vi "data_calibrate_and_grid.vi"(6 "Reset":bool=TRUE, 8 "Tare":bool=TRUE, 9 "Row Length":i32=64, 10 "No. Nodes":i32=64, 11 "Sensor Readings (PACKET)":i16[](array[numeric])) -> (0 "Node XYZ List":dbl[][](array[numeric]), 1 "Y (GRID)":dbl[][](array[numeric]), 2 "X (GRID)":dbl[][](array[numeric]), 3 "Z (GRID)":dbl[][](array[numeric]), 4 "Mag_GRID":dbl[][](array[numeric]))   [LabVIEW 2018]
panel:
  in  "Position Gain":dbl[](array[numeric])=[0.005, 0.005, 0.001]
  in  "Y Coords":dbl[](array[numeric])=[0.0, 15.0, 30.0, 45.0, 60.0, 75.0, 90.0, 105.0]
  in  "X Coords":dbl[](array[numeric])=[0.0, 15.0, 30.0, 45.0, 60.0, 75.0, 90.0, 105.0]
  in  "Tab Control":enum32{"16 Node", "64 Node"}(tab)=enum."64 Node"
  in  "Lookup Index n16":i32[](array[numeric])=[0, 2, 1, 3, 4, 6, 5, 7, 8, 10, 9, 11, 12, 14, 13, 15]
  in  "Inv Gain n16":i32[][](array[numeric])=[[1, 1, 1], [1, 1, -1], [1, 1, 1], [1, 1, 1], [1, 1, 1], [1, 1, -1], [1, 1, -1], [1, 1, -1], [1, 1, -1], [1, 1, -1], [1, 1, -1], [1, 1, 1], [1, 1, -1], [1, 1, 1], [1, 1, 1], [1, 1, -1]]
  in  "Lookup Index n64":i32[](array[numeric])=[0, 1, 2, 3, 4, 5, 6, 7, 15, 14, 13, 12, 11, 10, 9, 8, 16, 17, 18, 19, 20, 21, 22, 23, 31, 29, 30, 28, 27, 26, 25, 24, 32, 33, 34, 35, 36, 37, 38, 39, 47, 46, 45, 44, 43, 42, 41, 40, 55, 54, 53, 52, 51, 50, 49, 48, 63, 62, 61, 60, 59, 58, 57, 56]
  in  "Inv Gain n64":i32[][](array[numeric])=[[1, 1, 1], [1, 1, 1], [1, 1, 1], [1, 1, 1], [1, 1, 1], [1, 1, 1], [1, 1, 1], [1, 1, 1], [1, 1, 1], [1, 1, 1], [1, 1, 1], [1, 1, 1], [1, 1, 1], [1, 1, 1], [1, 1, 1], [1, 1, 1], [1, 1, 1], [1, 1, 1], [1, 1, 1], [1, 1, 1], [1, 1, 1], [1, 1, 1], [1, 1, 1], [1, 1, 1], [1, 1, 1], [1, 1, 1], [1, 1, -1], [1, 1, 1], [1, 1, 1], [1, 1, 1], [1, 1, 1], [1, 1, 1], [1, 1, 1], [1, 1, 1], [1, 1, 1], [1, 1, 1], [1, 1, 1], [1, 1, 1], [1, 1, 1], [1, 1, 1], [1, 1, 1], [1, 1, 1], [1, 1, 1], [1, 1, 1], [1, 1, 1], [1, 1, 1], [1, 1, 1], [1, 1, 1], [1, 1, 1], [1, 1, 1], [1, 1, 1], [1, 1, 1], [1, 1, 1], [1, 1, 1], [1, 1, 1], [1, 1, 1], [1, 1, 1], [1, 1, 1], [1, 1, 1], [1, 1, -1], [1, 1, -1], [1, 1, 1], [1, 1, 1], [1, 1, 1]]
  in  "Tare":dbl[][](array[numeric])=[[0.00018775, -0.000174232, 3312.98], [0.000139686, -0.00039953199999999997, 2906.42], [-0.000288384, -0.001229387, 2606.34], [-3.6799e-05, -0.0012016, 3702.6], [0.000266605, -0.001108476, 3847.7999999999997], [0.00038301, -0.000208027, 3472.7], [-0.000177236, -0.000316171, 3651.7799999999997], [-0.00024557699999999997, 0.000544475, 4767.4], [-5.6325e-05, -0.00041305, 4172.08], [8.4112e-05, 0.000956774, 2562.7799999999997], [-0.000261348, 0.001097962, 3675.98], [-0.00014944899999999998, -0.00066839, 4856.94], [-0.000204272, 0.000920726, 4740.78], [-0.000242573, -7.7353e-05, 4009.94], [0.000246328, -0.000138184, 4358.42], [7.51e-06, 0.000451351, 5829.78]]
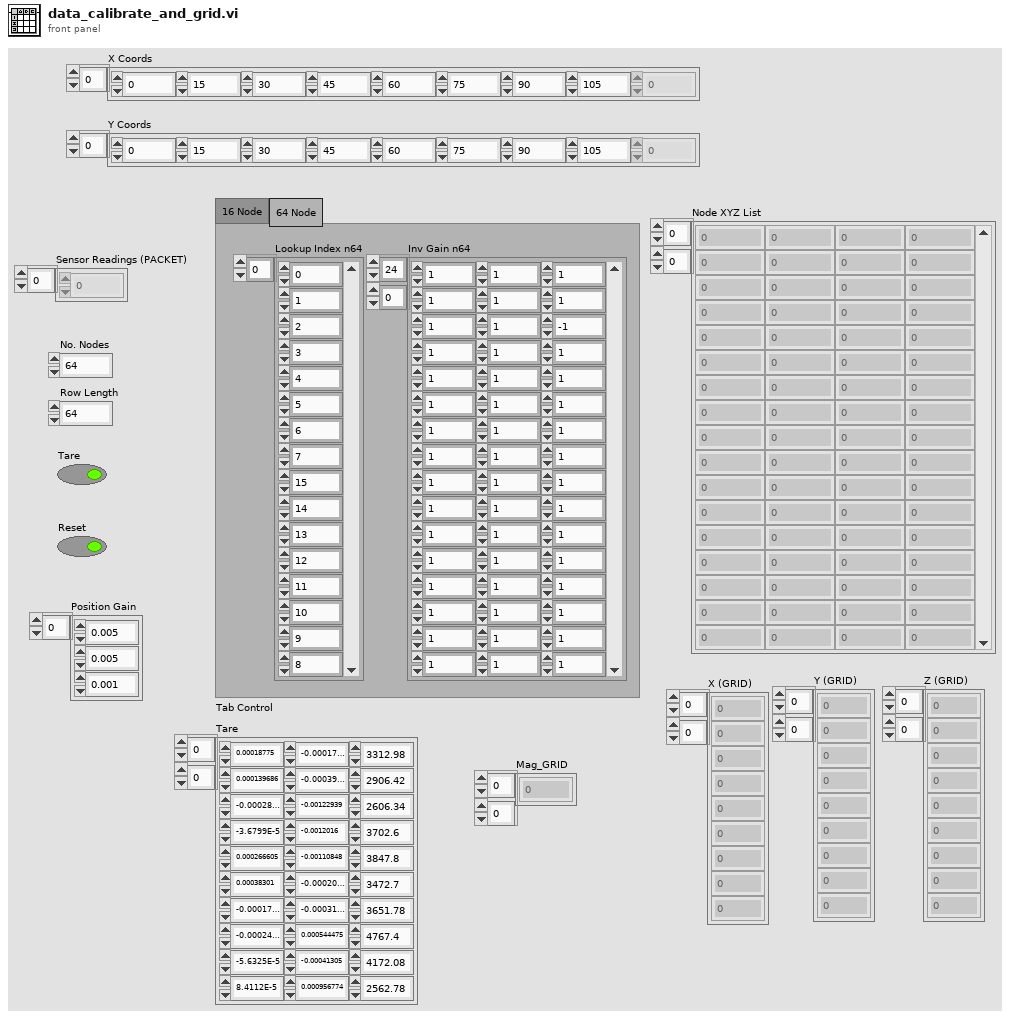
[diagram p1: front panel]
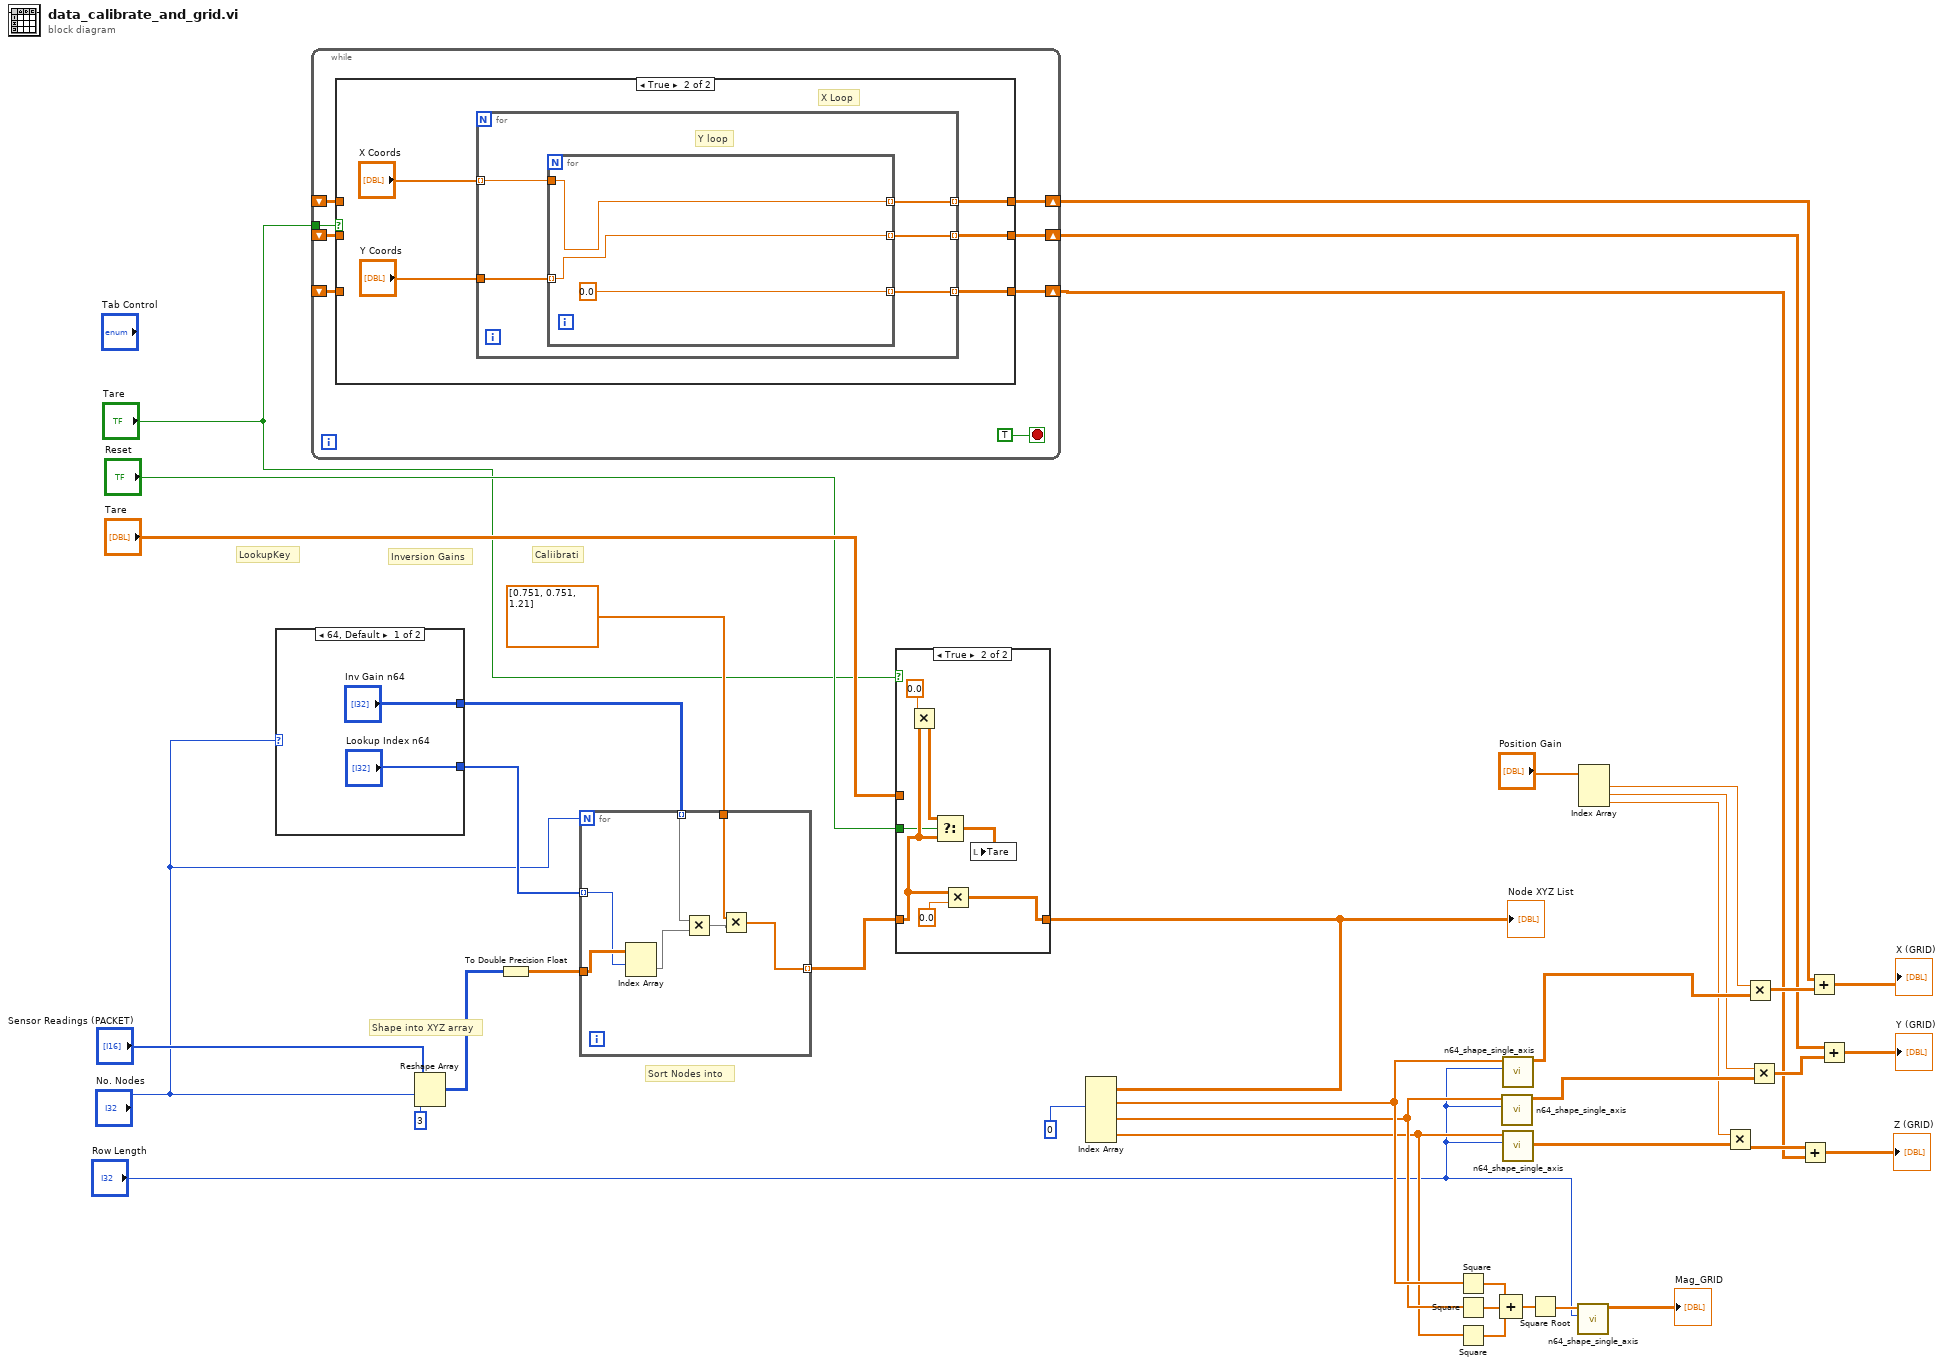
[diagram p0: block diagram]
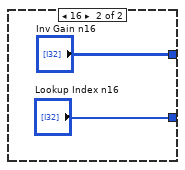
[diagram p3: hidden frame]
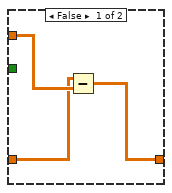
[diagram p4: hidden frame]
diagram:
  # "Caliibrati"
  # "Inversion Gains"
  # "LookupKey"
  # "Sort Nodes into"
  # "Shape into XYZ array"
  n1 = case shown="64, Default" "No. Nodes" {
    tunnel: ["Lookup Index n64" "Lookup Index n16"] -> w37
    tunnel: ["Inv Gain n64" "Inv Gain n16"] -> w35
    frame 64, Default {
    }
    frame 16 {
    }
  }
  n2 = while {
    tunnel: "Tare" -> [w52]
    shift-right: [w50] -> w12
    shift-left: _ -> [w47]
    shift-right: [w49] -> w9
    shift-left: _ -> [w46]
    shift-right: [w48] -> w2
    shift-left: _ -> [w45]
    stop <- TRUE stop-if-true
    n3 = case shown="True" w52 {
      tunnel: [w55 w58] -> w50
      tunnel: [w54 w57] -> w49
      tunnel: [w53 w56] -> w48
      tunnel: w47 -> [w55 _]
      tunnel: w46 -> [w54 _]
      tunnel: w45 -> [w53 _]
      frame False {
      }
      frame True {
        # "X Loop"
        n4 = for {
          tunnel: "X Coords" -> [w65] mode=indexing
          tunnel: "Y Coords" -> [w64]
          tunnel: [w63] -> w58 mode=indexing
          tunnel: [w62] -> w56 mode=indexing
          tunnel: [w61] -> w57 mode=indexing
          # "Y loop"
          n5 = for {
            tunnel: w65 -> [w68]
            tunnel: w64 -> [w66] mode=indexing
            tunnel: [w68] -> w63 mode=indexing
            tunnel: [0.0 ("element")] -> w62 mode=indexing
            tunnel: [w66] -> w61 mode=indexing
          }
        }
      }
    }
  }
  n6 = Reshape Array("Sensor Readings (PACKET)", "No. Nodes", 3 ("milliseconds to wait")) -> (w34:i16[][])
  n7 = To Double Precision Float(number=w34) -> (double precision float=w33:dbl[][])
  n8 = for {
    N: "No. Nodes" -> [_]
    tunnel: w33 -> [w75]
    tunnel: w37 -> [w69] mode=indexing
    tunnel: [w70] -> w32 mode=indexing
    tunnel: dbl[] [0.751, 0.751, 1.21] -> [w72]
    tunnel: w35 -> [w74] mode=indexing
    n9 = Index Array(array=w75, index (row)=w69) -> (element=w71:dbl[])  [unwired: 1 in]
    n10 = Multiply(x=w74, y=w71) -> (x*y=w73:dbl[])
    n11 = Multiply(x=w72, y=w73) -> (x*y=w70:dbl[])
  }
  n12 = case shown="True" "Tare" {
    tunnel: w32 -> [w76 w82]
    tunnel: [w78 w84] -> w31
    tunnel: "Tare" -> [w77 _]
    tunnel: "Reset" -> [_ w79]
    frame False {
      n13 = Subtract(x=w76, y=w77) -> (x-y=w78:dbl[][])
    }
    frame True {
      n14 = Multiply(x=0.0 ("milliseconds to wait"), y=w82) -> (x*y=w81:dbl[][])
      n15 = Select(t=w81, s=w79, f=w82) -> (s? t:f=w83:dbl[][])
      n16 = Multiply(x=w82, y=0.0 ("milliseconds to wait")) -> (x*y=w84:dbl[][])
      n17 = local write "Tare"(w83) -> ()
    }
  }
  "Node XYZ List" <- w31
  n18 = Index Array(array=w31, index (col) #1=0 ("disabled index (col)")) -> (element #1=w28:dbl[], element #2=w27:dbl[], element #3=w26:dbl[])  [unwired: 5 in]
  n19 = Square(x=w28) -> (x^2=w25:dbl[])
  n20 = Square(x=w27) -> (x^2=w23:dbl[])
  n21 = Square(x=w26) -> (x^2=w24:dbl[])
  n22 = Compound Arithmetic op=ADD(w25, w23, w24) -> (w22:dbl[])
  n23 = call "n64_shape_single_axis.vi"("Row Length"="Row Length", "Readings (FLAT)"=w27) -> ("Readings (GRID)"=w8:dbl[][])  [unwired: 9 in]
  n24 = call "n64_shape_single_axis.vi"("Row Length"="Row Length", "Readings (FLAT)"=w28) -> ("Readings (GRID)"=w17:dbl[][])  [unwired: 9 in]
  n25 = call "n64_shape_single_axis.vi"("Row Length"="Row Length", "Readings (FLAT)"=w26) -> ("Readings (GRID)"=w5:dbl[][])  [unwired: 9 in]
  n26 = Square Root(x=w22) -> (sqrt(x)=w21:dbl[])
  n27 = call "n64_shape_single_axis.vi"("Row Length"="Row Length", "Readings (FLAT)"=w21) -> ("Readings (GRID)"=→"Mag_GRID":dbl[][])  [unwired: 9 in]
  n28 = Index Array(array="Position Gain") -> (element #1=w13:dbl, element #2=w11:dbl, element #3=w4:dbl)  [unwired: 3 in]
  n29 = Multiply(x=w4, y=w5) -> (x*y=w3:dbl[][])
  n30 = Multiply(x=w13, y=w17) -> (x*y=w15:dbl[][])
  n31 = Multiply(x=w11, y=w8) -> (x*y=w10:dbl[][])
  n32 = Add(x=w3, y=w2) -> (x+y=→"Z (GRID)":dbl[][])
  n33 = Add(x=w12, y=w15) -> (x+y=→"X (GRID)":dbl[][])
  n34 = Add(x=w9, y=w10) -> (x+y=→"Y (GRID)":dbl[][])
